vi "Request Room Details.vi"(0 "Rooms Manager UI in":refnum<class "Rooms Manager UI.lvclass">, 5 "Row":i32, 7 "Column":i32, 11 "error in (no error)":errorcluster) -> (4 "Rooms Manager UI out":refnum<class "Rooms Manager UI.lvclass">, 15 "error out":errorcluster)   [LabVIEW 2023, in "Rooms Manager UI.lvlib" / "Rooms Manager UI.lvclass"]
uses:
  Rooms Manager UI.lvclass
  <vilib>/ActorFramework/Actor/Actor.lvclass/Actor.ctl
  Rooms Manager UI.lvclass/Rooms Manager UI.ctl
  Rooms Manager UI Messages/Refresh Active Room Details Msg/Refresh Active Room Details Msg.lvclass/Refresh Active Room Details Msg.ctl
  <vilib>/ActorFramework/Message Enqueuer/Message Enqueuer.lvclass/Message Enqueuer.ctl
  <vilib>/ActorFramework/Message Enqueuer/Enqueue.vi
  Rooms Manager UI Messages/Refresh Active Room Details Msg/Refresh Active Room Details Msg.lvclass
  <vilib>/ActorFramework/Message Priority Queue/Priority Enqueue.vi
  <vilib>/ActorFramework/Actor/Actor.lvclass
  Utilities/Utilities.lvlib
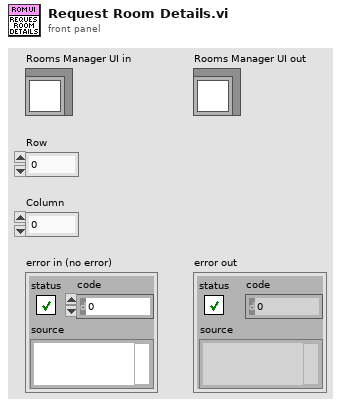
[diagram p1: front panel]
types:
  T1 = cluster{"Room No":string, "Alert":bool, "Occupied":bool, "Maintainance":bool, "IsActive":bool}[][]
  T2 = cluster{"Room No":string, "Alert":bool, "Occupied":bool, "Maintainance":bool, "IsActive":bool}
  T3 = enum8{"Enabled", "Disabled", "Disabled and Grayed Out"}
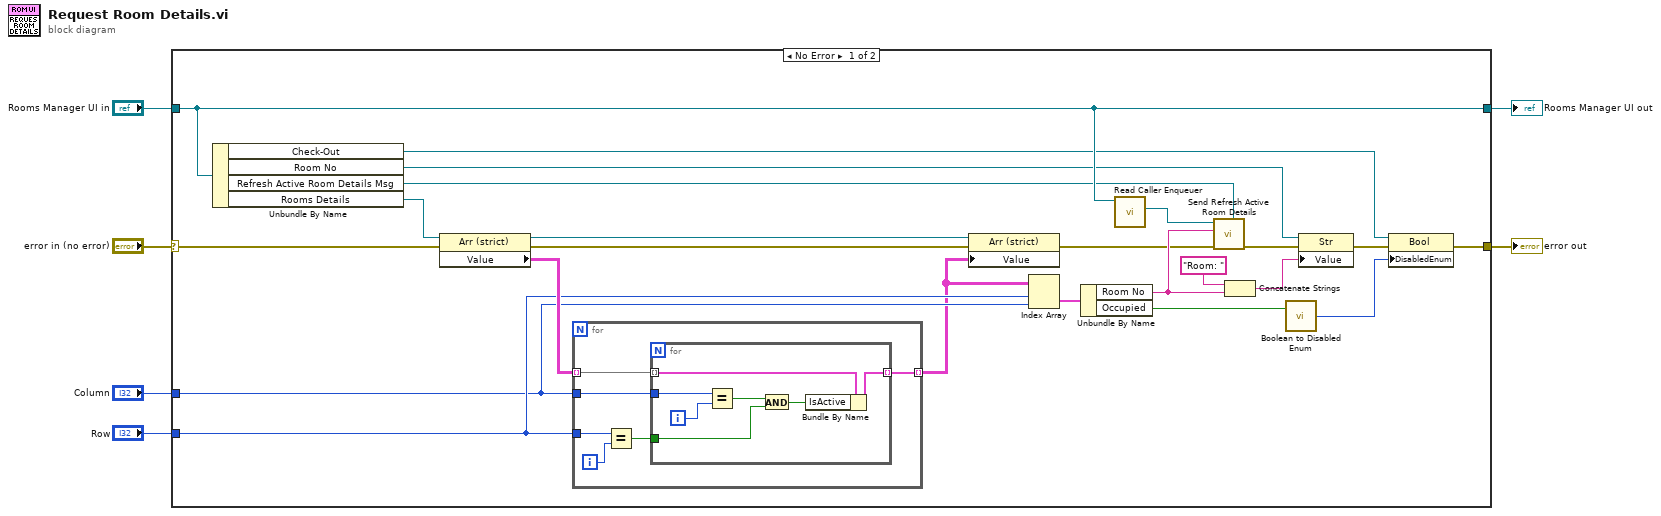
[diagram p0: block diagram]
diagram:
  n1 = case shown="No Error" "error in (no error)" {
    selector: "error in (no error)" -> [w29 w44]
    tunnel: [w10 w44] -> w5
    tunnel: [w25 w43] -> w3
    tunnel: "Rooms Manager UI in" -> [w25 w43]
    tunnel: "Row" -> [w13 _]
    tunnel: "Column" -> [w12 _]
    frame No Error {
      n2 = Unbundle By Name(w25) -> ("Check-Out"=w9:refnum<vi>, "Room No"=w21:refnum<vi>, "Refresh Active Room Details Msg"=w23:refnum<class "Refresh Active Room Details Msg.lvclass">, "Rooms Details"=w28:refnum<vi>)
      n3 = property class="Arr (strict)"(reference=w28, error in=w29) -> (reference out=w17:refnum<vi>, error out=w16:errorcluster, "Value"=w14:T1)
      n4 = for {
        tunnel: w14 -> [w35] mode=indexing
        tunnel: w13 -> [w33]
        tunnel: w12 -> [w34]
        tunnel: [w30] -> w11 mode=indexing
        i -> [w32]
        n5 = Equal?(x=w33, y=w32) -> (x = y?=w31:bool)
        n6 = for {
          tunnel: w35 -> [w42] mode=indexing
          tunnel: w34 -> [w41]
          tunnel: w31 -> [w39]
          tunnel: [w36] -> w30 mode=indexing
          i -> [w40]
          n7 = Equal?(x=w41, y=w40) -> (x = y?=w38:bool)
          n8 = And(x=w38, y=w39) -> (x .and. y?=w37:bool)
          n9 = Bundle By Name(cluster=w42, "IsActive"=w37) -> (w36:T2)
        }
      }
      n10 = property class="Arr (strict)"(reference=w17, error in=w16, "Value"=w11) -> (error out=w15:errorcluster)  [unwired: 1 out]
      n11 = Index Array(array=w11, index (row)=w13, index (col)=w12) -> (element=w27:T2)
      n12 = Unbundle By Name(w27) -> ("Room No"=w20:string, "Occupied"=w8:bool)
      n13 = call <vilib>:"Read Caller Enqueuer.vi"("Actor"=w25) -> ("Caller Enqueuer"=w24:refnum<class "Message Enqueuer.lvclass">)  [unwired: 10 in]
      n14 = call "Send Refresh Active Room Details.vi"("Message Type"=w23, "error in (no error)"=w15, "Active Room"=w20, "Message Enqueuer"=w24) -> ("error out"=w26:errorcluster)  [unwired: 6 in, 1 out]
      n15 = Concatenate Strings("Room: ", w20) -> (w19:string)
      n16 = call "Boolean to Disabled Enum.vi"("Enable"=w8) -> ("Disabled"=w7:T3)  [unwired: 1 in]
      n17 = property class="Str"(reference=w21, error in=w26, "Value"=w19) -> (error out=w22:errorcluster)  [unwired: 1 out]
      n18 = property class="Bool"(reference=w9, error in=w22, "DisabledEnum"=w7) -> (error out=w10:errorcluster)  [unwired: 1 out]
    }
    frame Error {
    }
  }
  "error out" <- w5
  "Rooms Manager UI out" <- w3
